vi "Handle Error.vi"(8 "error in (no error)":errorcluster, 11 "Configuration in":refnum<class "Configuration.lvclass">) -> (0 "error out":errorcluster, 2 "stop actor?":bool=TRUE, 3 "Configuration out":refnum<class "Configuration.lvclass">)   [LabVIEW 2016, in "Configuration.lvlib" / "Configuration.lvclass"]
doc: "(<B>Filename</B>: Actor Framework.lvlib:Actor.lvclass:Handle Error.vi)\n\nDefines how the actor handles an error that occurred while processing a message. By default, this method does nothing except stop the actor."
uses:
  <userlib>/Configuration Dialog Actor/Configuration.lvclass
  C:/Program Files (x86)/National Instruments/LabVIEW 2016/vi.lib/ActorFramework/Actor/Actor.lvclass
  <vilib>/ActorFramework/Actor/Actor.lvclass/Actor.ctl
  <userlib>/Common Components/Function Messages/Log in MsgList Msg/Log in MsgList Msg.lvclass/Log in MsgList Msg.ctl
  <vilib>/ActorFramework/Message Enqueuer/Message Enqueuer.lvclass/Message Enqueuer.ctl
  <vilib>/ActorFramework/Message Enqueuer/Enqueue.vi
  <userlib>/Common Components/Function Messages/Log in MsgList Msg/Log in MsgList Msg.lvclass
  C:/Program Files (x86)/National Instruments/LabVIEW 2016/vi.lib/ActorFramework/Message/Message.lvclass
  <vilib>/ActorFramework/Message Priority Queue/Priority Enqueue.vi
  <vilib>/ActorFramework/Actor/Actor.lvclass
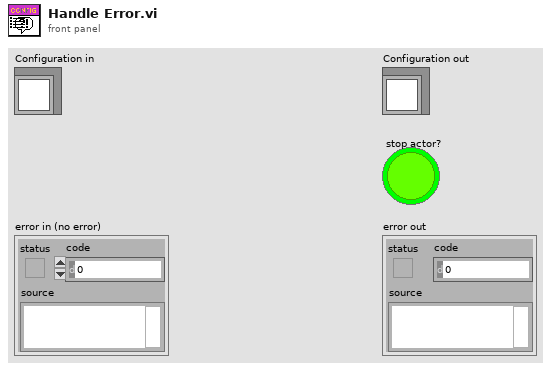
[diagram p1: front panel]
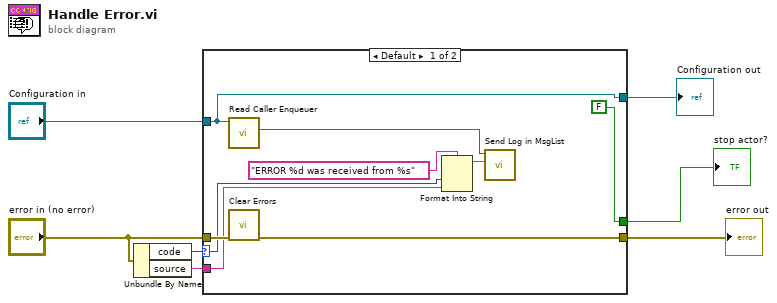
[diagram p0: block diagram]
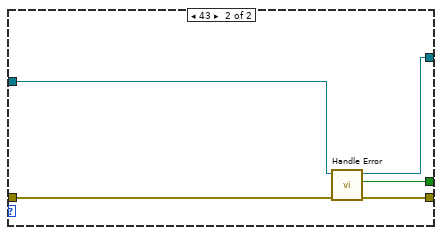
[diagram p2: hidden frame]
diagram:
  n1 = Unbundle By Name("error in (no error)") -> ("code"=w2:i32, "source"=w1:string)
  n2 = case shown="Default" w2 {
    selector: w2 -> [w11 _]
    tunnel: [w13 w21] -> w7
    tunnel: [FALSE ("stop actor?") w20] -> w6
    tunnel: [w8 w19] -> w5
    tunnel: "Configuration in" -> [w8 w18]
    tunnel: "error in (no error)" -> [w14 w17]
    tunnel: w1 -> [w10 _]
    frame Default {
      n3 = call <vilib>:"Read Caller Enqueuer.vi"("Actor"=w8) -> ("Caller Enqueuer"=w9:refnum<class "Message Enqueuer.lvclass">)  [unwired: 10 in]
      n4 = call <vilib>:"Clear Errors.vi"("error in (no error)"=w14) -> ("error out"=w13:errorcluster)  [unwired: 5 in, 1 out]
      n5 = Format Into String(format string="ERROR %d was received from %s", w11, w10) -> (resulting string=w15:string)  [unwired: 2 in, 1 out]
      n6 = call <userlib>:"Send Log in MsgList.vi"("Msg"=w15, "Message Enqueuer"=w9) -> ()  [unwired: 8 in, 2 out]
    }
    frame 43 {
      n7 = call-parent "Handle Error.vi"("error in (no error)"=w17, "Actor in"=w18) -> ("error out"=w21:errorcluster, "stop actor?"=w20:bool, "Actor out"=w19:refnum<class "Configuration.lvclass">)  [unwired: 7 in]
    }
  }
  "Configuration out" <- w5
  "error out" <- w7
  "stop actor?" <- w6
